vi "Test shm monitor Command standby LV.vi"(8 "error in (no error)":errorcluster, 11 "command_standby_Ctl":cluster{"value":u8}) -> (0 "error out":errorcluster, 2 "function return":i32, 3 "command_standby_Ctl out":cluster{"value":u8})   [LabVIEW 2018, in "SALLV_Test.lvlib"]
doc: "int Test_shm_monitorCommand_standbyLV(Test_command_standbyLV *command_standby_Ctl );"
uses:
  SALLV_Test.lvlib
  SALLV_Test.so
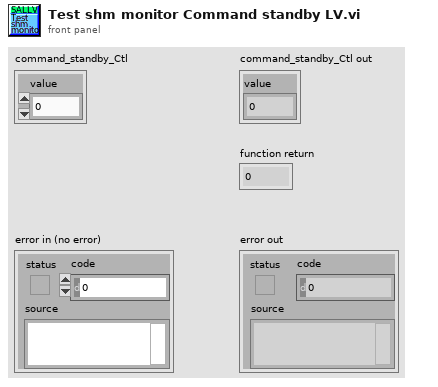
[diagram p1: front panel]
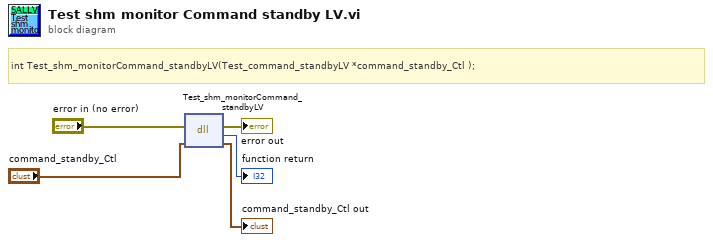
[diagram p0: block diagram]
diagram:
  # "int Test_shm_monitorCommand_standbyLV(Test_command_standbyLV *command_standby_Ctl );"
  n1 = dll-call lib="home/ttsai/Documents/salLabVIEWtestData/SALLV_Test.*" fn="Test_shm_monitorCommand_standbyLV"(error in="error in (no error)", "command_standby_Ctl"="command_standby_Ctl") -> (error out=→"error out":errorcluster, →"function return":i32, "command_standby_Ctl"=→"command_standby_Ctl out":cluster{"value":u8})  [unwired: 2 in, 1 out]
